vi "Quick Usb Read Default.vi"(8 "error in (no error)":errorcluster, 9 "data":u16, 10 "address":u16, 11 "hDevice":u32) -> (0 "error out":errorcluster, 1 "data out":u16, 2 "function return":i32, 3 "hDevice out":u32)   [LabVIEW 2011, in "QuickUSB.lvlib"]
doc: "QUSBLIB QRETURN QuickUsbReadDefault(\n QHANDLE hDevice,\n QWORD address, \n PQWORD data\n);"
uses:
  QuickUSB.lvlib
  QuickUSB.dll
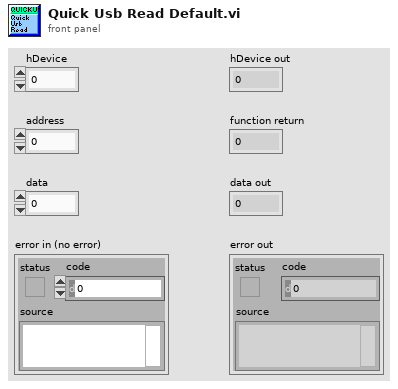
[diagram p1: front panel]
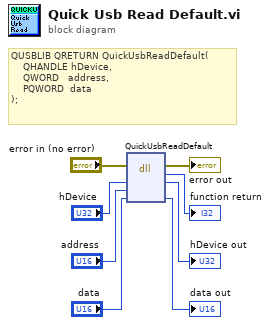
[diagram p0: block diagram]
diagram:
  # "QUSBLIB QRETURN QuickUsbReadDefault(\n    QHANDLE hDevice,\n    QWORD   address, \n    PQWORD  data\n);"
  n1 = dll-call lib="C:/QuickUSB/QuickUSB.*" fn="QuickUsbReadDefault"(error in="error in (no error)", "hDevice"="hDevice", "address"="address", "data"="data") -> (error out=→"error out":errorcluster, →"function return":i32, "hDevice"=→"hDevice out":u32, "data"=→"data out":u16)  [unwired: 3 in, 1 out]
